vi "NI DOCO DEMO_Same Sample_OK.vi"() -> ()   [LabVIEW 2018]
uses:
  <vilib>/DAQmx/write.llb/DAQmx Write (Digital 1D Wfm NChan NSamp).vi
  <vilib>/DAQmx/write.llb/DAQmx Write (Analog 1D Wfm NChan NSamp).vi
  <vilib>/DAQmx/create/channels.llb/DAQmx Create Channel (AO-Voltage-Basic).vi
  <vilib>/DAQmx/configure/timing.llb/DAQmx Timing (Sample Clock).vi
  <vilib>/Waveform/WDTOps.llb/WDT Number of Waveform Samples DBL.vi
  <vilib>/Waveform/WDTOps.llb/WDT Append Waveforms DBL.vi
  <vilib>/DAQmx/miscellaneous.llb/DAQmx Fill In Error Info.vi
  <vilib>/Waveform/DTblOps.llb/DTbl Digital to Boolean Array.vi
  <vilib>/DAQmx/create/channels.llb/DAQmx Create Channel (DO-Digital Output).vi
  <vilib>/Waveform/DWDTOps.llb/DWDT Uncompress Digital.vi
  <vilib>/Waveform/DWDTOps.llb/DWDT Append Digital Samples.vi
  <resource>/objmgr/daqmx.rc
panel:
  out "DO size 3":i32
  out "DO size 2":i32
  out "DO size":i32
  out "number of samples 3":i32
  out "number of samples 2":i32
  out "number of samples":i32
  out "Mixed Signal Graph 2":cluster{waveform(dbl)[], digitalwaveform[]}(graph)
  out "Mixed Signal Graph":cluster{waveform(dbl)[], digitalwaveform[]}(graph)
  out "initialized array":digitalwaveform[](array[waveform])
  out "Waveform Graph":waveform(dbl)[](graph)
  out "Digital Waveform Graph":digitalwaveform[](graph)
  out "size(s) 4":i32
  out "size(s) 3":i32
  out "size(s) 2":i32
  out "size(s)":i32
  out "NumChans 2":u32
  out "NumChans":u32
  out "Numeric":u32
  in  "Enum":enum16{"A A", "A B", "B B", "B A"}(ring)=enum."A B"
  in  "stop 2":bool
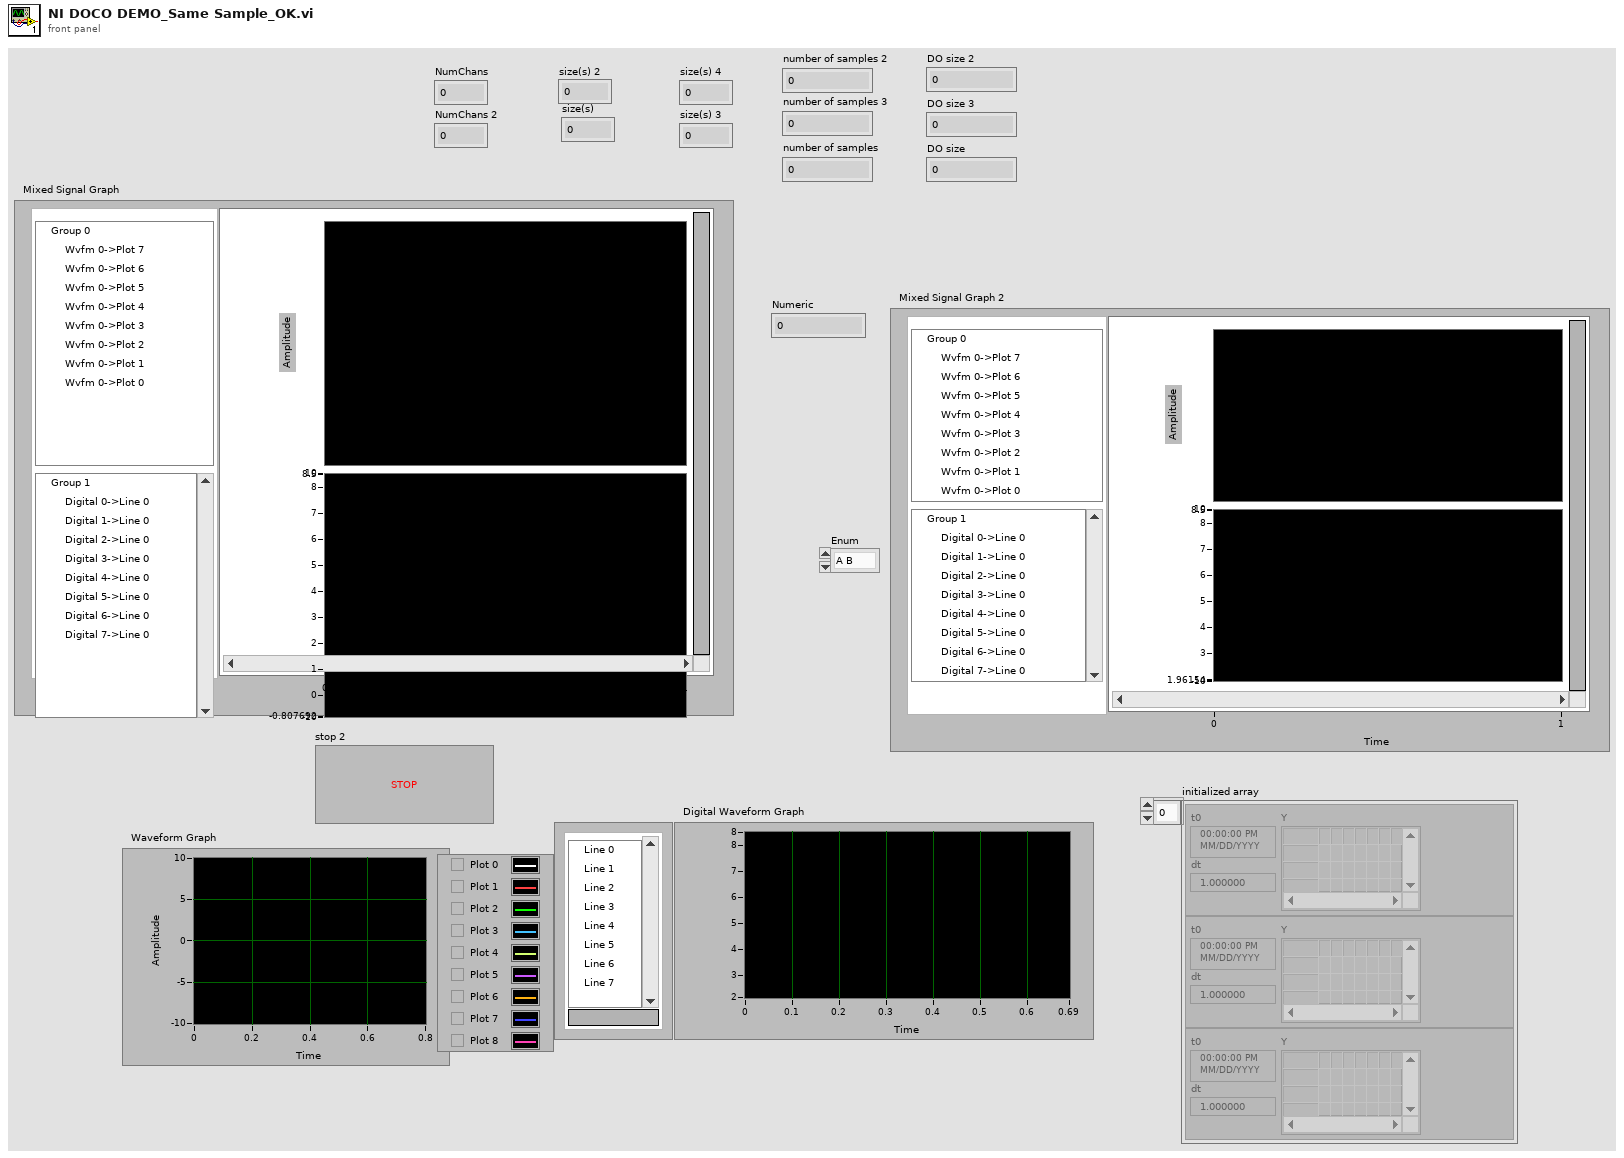
[diagram p1: front panel]
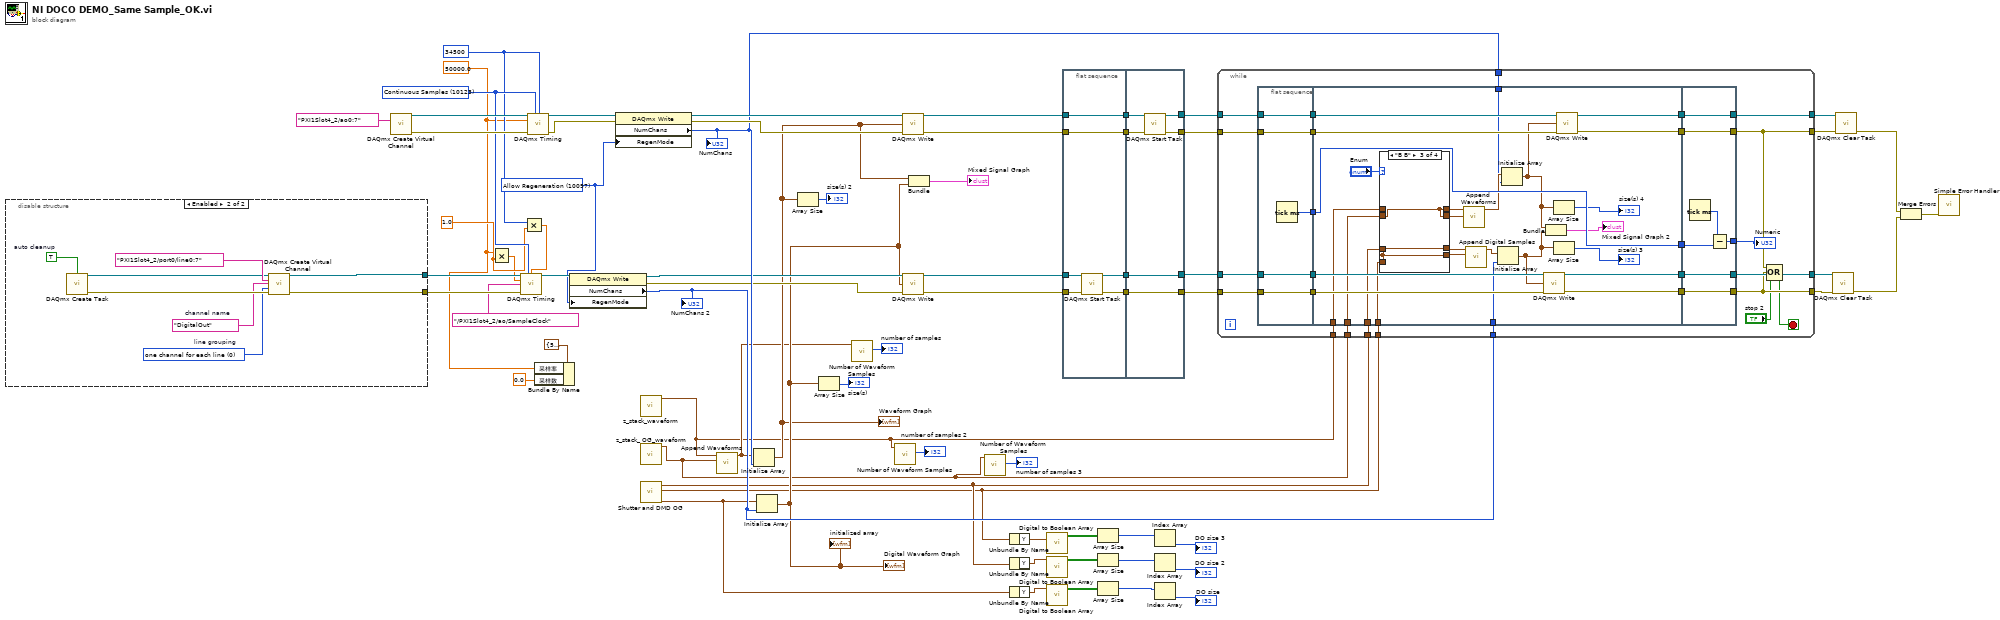
[diagram p0: block diagram]
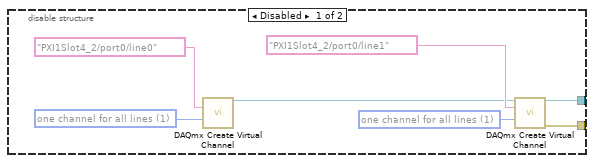
[diagram p2: hidden frame]
diagram:
  w27 = 1.0 ("y")
  w30 = 10097 items=["Allow Regeneration"=10097, "Do Not Allow Regeneration"=10158] ("RegenMode")
  w29 = 34500 ("samples per channel")
  w64 = 10123 items=["Finite Samples"=10178, "Continuous Samples"=10123, "Hardware Timed Single Point"=12522] ("sample mode")
  w2 = 50000.0 ("rate")
  n1 = disable-structure shown="Enabled" {
    disable-tunnel: [w75 w77] -> w66
    disable-tunnel: [w74 w78] -> w65
    frame Disabled {
      w70 = 1 items=["one channel for each line", "one channel for all lines"] ("line grouping")
      w73 = 1 items=["one channel for each line", "one channel for all lines"] ("line grouping")
      n2 = call-poly <vilib>:"DAQmx Create Virtual Channel.vi"("lines"=tag "PXI1Slot4_2/port0/line0", "line grouping"=w70) -> ("task out"=w71:refnum<k21>)  [unwired: 12 in, 1 out]
      n3 = call-poly <vilib>:"DAQmx Create Virtual Channel.vi"("task in"=w71, "lines"=tag "PXI1Slot4_2/port0/line1", "line grouping"=w73) -> ("task out"=w74:refnum<k21>, "error out"=w75:errorcluster)  [unwired: 11 in]
    }
    frame Enabled {
      w79 = TRUE  # auto cleanup
      w83 = 0 items=["one channel for each line", "one channel for all lines"]  # line grouping
      w82 = "DigitalOut"  # channel name
      n4 = call <vilib>:"DAQmx Create Task.vi"("auto cleanup"=w79) -> ("task out"=w80:refnum<k21>, "error out"=w84:errorcluster)  [unwired: 13 in]
      n5 = call-poly <vilib>:"DAQmx Create Virtual Channel.vi"("task in"=w80, "lines"=tag "PXI1Slot4_2/port0/line0:7", "name to assign"=w82, "line grouping"=w83, "error in"=w84) -> ("task out"=w78:refnum<k21>, "error out"=w77:errorcluster)  [unwired: 9 in]
    }
  }
  n6 = call-poly <vilib>:"DAQmx Create Virtual Channel.vi"("physical channels"=tag "PXI1Slot4_2/ao0:7") -> ("task out"=w68:refnum<k21>, "error out"=w67:errorcluster)  [unwired: 13 in]
  n7 = Multiply(x=w2, y=w27) -> (x*y=w4:dbl)
  n8 = Multiply(x=w29, y=w27) -> (x*y=w28:dbl)
  n9 = call-poly <vilib>:"DAQmx Timing.vi"("task/channels in"=w65, "sample mode"=w64, "samples per channel"=w28, "rate"=w4, "source"=tag "/PXI1Slot4_2/ao/SampleClock", "error in"=w66) -> ("task out"=w38:refnum<k21>)  [unwired: 8 in, 1 out]
  n10 = call-poly <vilib>:"DAQmx Timing.vi"("task/channels in"=w68, "sample mode"=w64, "samples per channel"=w29, "rate"=w2, "error in"=w67) -> ("task out"=w43:refnum<k21>, "error out"=w42:errorcluster)  [unwired: 9 in]
  n11 = Bundle By Name(cluster=cluster{"采样率":dbl, "采样数":dbl} {"采样率"=500000.0, "采样数"=130000.0} ("Z stack acquisition 采样信息"), "采样率"=w2, "采样数"=0.0) -> ()  [unwired: 1 out]
  n12 = property class="DAQmx Write"(reference=w38, "RegenMode"=w30) -> (reference out=w37:refnum<k21>, error out=w36:errorcluster, "NumChans"=w35:u32)  [unwired: 1 in]
  "NumChans 2" <- w35
  n13 = property class="DAQmx Write"(reference=w43, error in=w42, "RegenMode"=w30) -> (reference out=w41:refnum<k21>, error out=w40:errorcluster, "NumChans"=w39:u32)
  "NumChans" <- w39
  n14 = call "z_stack_waveform.vi"() -> ("waveform out"=w23:waveform(dbl))  [unwired: 9 in, 2 out]
  n15 = call "z_stack_ OG_waveform.vi"() -> ("waveform out"=w21:waveform(dbl))  [unwired: 15 in, 4 out]
  n16 = call "Shutter and DMD OG.vi"() -> ("output waveform"=w19:digitalwaveform, "output waveform 2"=w9:digitalwaveform, "output waveform1"=w10:digitalwaveform)  [unwired: 8 in]
  n17 = call-poly <vilib>:"Append Waveforms.vi"("waveform B"=w21, "waveform A"=w23) -> ("waveform out"=w24:waveform(dbl))  [unwired: 8 in, 1 out]
  n18 = Initialize Array(w24, w39) -> (w26:waveform(dbl)[])
  "Waveform Graph" <- w26
  n19 = Initialize Array(w19, w35) -> (w32:digitalwaveform[])
  "Digital Waveform Graph" <- w32
  "initialized array" <- w32
  n20 = Array Size(array=w26) -> (size(s)=→"size(s) 2":i32)
  n21 = Array Size(array=w32) -> (size(s)=→"size(s)":i32)
  n22 = call-poly <vilib>:"Number of Waveform Samples.vi"("waveform in"=w24) -> ("number of samples"=→"number of samples":i32)  [unwired: 8 in, 2 out]
  n23 = call-poly <vilib>:"Number of Waveform Samples.vi"("waveform in"=w23) -> ("number of samples"=→"number of samples 2":i32)  [unwired: 8 in, 2 out]
  n24 = call-poly <vilib>:"DAQmx Write.vi"("task/channels in"=w41, "data"=w26, "error in"=w40) -> ("task out"=w62:refnum<k21>, "error out"=w58:errorcluster)  [unwired: 10 in, 1 out]
  n25 = call-poly <vilib>:"DAQmx Write.vi"("task/channels in"=w37, "data"=w32, "error in"=w36) -> ("task out"=w45:refnum<k21>, "error out"=w44:errorcluster)  [unwired: 10 in, 1 out]
  n26 = Bundle(w26, w32) -> (→"Mixed Signal Graph":cluster{waveform(dbl)[], digitalwaveform[]})  [unwired: 1 in]
  n27 = call-poly <vilib>:"Number of Waveform Samples.vi"("waveform in"=w21) -> ("number of samples"=→"number of samples 3":i32)  [unwired: 8 in, 2 out]
  n28 = Unbundle By Name(w9) -> ("Y"=w13:digitaldata)
  n29 = Unbundle By Name(w10) -> ("Y"=w11:digitaldata)
  n30 = Unbundle By Name(w19) -> ("Y"=w14:digitaldata)
  n31 = call-poly <vilib>:"Digital to Boolean Array.vi"("digital data"=w13) -> ("boolean array"=w8:bool[][])  [unwired: 9 in, 1 out]
  n32 = call-poly <vilib>:"Digital to Boolean Array.vi"("digital data"=w11) -> ("boolean array"=w7:bool[][])  [unwired: 9 in, 1 out]
  n33 = call-poly <vilib>:"Digital to Boolean Array.vi"("digital data"=w14) -> ("boolean array"=w18:bool[][])  [unwired: 9 in, 1 out]
  n34 = flat-sequence {
    tunnel: w62 -> [w90]
    tunnel: w45 -> [w89]
    tunnel: w44 -> [w88]
    tunnel: [w90] -> w61
    tunnel: [w87] -> w60
    tunnel: [w86] -> w59
    tunnel: w58 -> [w85]
    tunnel: [w85] -> w57
    tunnel: w61 -> [w94]
    tunnel: [w96] -> w54
    tunnel: w60 -> [w96]
    tunnel: [w95] -> w53
    tunnel: w59 -> [w95]
    tunnel: [w93] -> w56
    tunnel: w57 -> [w92]
    tunnel: [w91] -> w55
    frame #0 {
      n35 = call <vilib>:"DAQmx Start Task.vi"("task/channels in"=w89, "error in"=w88) -> ("task out"=w87:refnum<k21>, "error out"=w86:errorcluster)  [unwired: 12 in]
    }
    frame #1 {
      n36 = call <vilib>:"DAQmx Start Task.vi"("task/channels in"=w94, "error in"=w92) -> ("task out"=w93:refnum<k21>, "error out"=w91:errorcluster)  [unwired: 12 in]
    }
  }
  n37 = Array Size(array=w8) -> (size(s)=w6:i32[])
  n38 = Array Size(array=w7) -> (size(s)=w5:i32[])
  n39 = Array Size(array=w18) -> (size(s)=w17:i32[])
  n40 = Index Array(array=w6) -> (element=→"DO size 3":i32)  [unwired: 1 in]
  n41 = Index Array(array=w5) -> (element=→"DO size 2":i32)  [unwired: 1 in]
  n42 = Index Array(array=w17) -> (element=→"DO size":i32)  [unwired: 1 in]
  n43 = while {
    tunnel: w56 -> [w121]
    tunnel: w55 -> [w120]
    tunnel: w54 -> [w123]
    tunnel: w53 -> [w122]
    tunnel: [w117] -> w51
    tunnel: [w119] -> w52
    tunnel: [w118] -> w50
    tunnel: [w116] -> w49
    tunnel: w23 -> [w113]
    tunnel: w21 -> [w112]
    tunnel: w10 -> [w111]
    tunnel: w9 -> [w110]
    tunnel: w39 -> [w98]
    tunnel: w35 -> [w97]
    stop <- w115 stop-if-true
    n44 = flat-sequence {
      tunnel: w120 -> [w125]
      tunnel: w121 -> [w126]
      tunnel: w122 -> [w127]
      tunnel: w123 -> [w128]
      tunnel: [w128] -> w109
      tunnel: [w127] -> w108
      tunnel: [w126] -> w107
      tunnel: [w125] -> w106
      tunnel: [w124] -> w101
      tunnel: w113 -> [w146]
      tunnel: w112 -> [w145]
      tunnel: w111 -> [w144]
      tunnel: w110 -> [w143]
      tunnel: w109 -> [w155]
      tunnel: w108 -> [w154]
      tunnel: w107 -> [w153]
      tunnel: w106 -> [w152]
      tunnel: [w151] -> w105
      tunnel: [w150] -> w104
      tunnel: [w149] -> w103
      tunnel: [w148] -> w102
      tunnel: w101 -> [w138]
      tunnel: [w138] -> w100
      tunnel: w98 -> [w136]
      tunnel: w97 -> [w134]
      tunnel: [w171] -> w116
      tunnel: [w172] -> w117
      tunnel: [w173] -> w118
      tunnel: [w174] -> w119
      tunnel: w105 -> [w174]
      tunnel: w104 -> [w173]
      tunnel: w103 -> [w172]
      tunnel: w102 -> [w171]
      tunnel: w100 -> [w169]
      tunnel: [w168] -> w99
      frame #0 {
        n45 = Tick Count (ms)() -> (millisecond timer value=w124:u32)
      }
      frame #1 {
        n46 = case shown="\"B B\"" "Enum" {
          tunnel: w146 -> [w157 w161 _ w166]
          tunnel: w145 -> [_ w160 w163 w167]
          tunnel: w144 -> [w156 w159 _ w164]
          tunnel: w143 -> [_ w158 w162 w165]
          tunnel: [w157 w161 w163 w167] -> w142
          tunnel: [w157 w160 w163 w166] -> w141
          tunnel: [w156 w159 w162 w165] -> w140
          tunnel: [w156 w158 w162 w164] -> w139
          frame "A A", Default {
          }
          frame "A B" {
          }
          frame "B B" {
          }
          frame "B A" {
          }
        }
        n47 = call-poly <vilib>:"Append Waveforms.vi"("waveform B"=w141, "waveform A"=w142) -> ("waveform out"=w137:waveform(dbl))  [unwired: 8 in, 1 out]
        n48 = call-poly <vilib>:"Append Digital Samples.vi"("digital waveform B"=w139, "digital waveform A"=w140) -> ("digital waveform out"=w135:digitalwaveform)  [unwired: 8 in, 1 out]
        n49 = Initialize Array(w135, w134) -> (w132:digitalwaveform[])
        n50 = Initialize Array(w137, w136) -> (w133:waveform(dbl)[])
        n51 = call-poly <vilib>:"DAQmx Write.vi"("task/channels in"=w155, "data"=w132, "error in"=w154) -> ("task out"=w150:refnum<k21>, "error out"=w148:errorcluster)  [unwired: 10 in, 1 out]
        n52 = Bundle(w133, w132) -> (→"Mixed Signal Graph 2":cluster{waveform(dbl)[], digitalwaveform[]})  [unwired: 1 in]
        n53 = Array Size(array=w133) -> (size(s)=→"size(s) 4":i32)
        n54 = Array Size(array=w132) -> (size(s)=→"size(s) 3":i32)
        n55 = call-poly <vilib>:"DAQmx Write.vi"("task/channels in"=w153, "data"=w133, "error in"=w152) -> ("task out"=w151:refnum<k21>, "error out"=w149:errorcluster)  [unwired: 10 in, 1 out]
      }
      frame #2 {
        n56 = Tick Count (ms)() -> (millisecond timer value=w170:u32)
        n57 = Subtract(x=w170, y=w169) -> (x-y=w168:u32)
      }
    }
    n58 = Compound Arithmetic op=OR(w117, w116, "stop 2") -> (w115:bool)
    "Numeric" <- w99
  }
  n59 = call <vilib>:"DAQmx Clear Task.vi"("task in"=w50, "error in"=w49) -> ("error out"=w47:errorcluster)  [unwired: 13 in]
  n60 = call <vilib>:"DAQmx Clear Task.vi"("task in"=w52, "error in"=w51) -> ("error out"=w48:errorcluster)  [unwired: 13 in]
  n61 = Merge Errors(w48, w47) -> (w46:errorcluster)
  n62 = call <vilib>:"Simple Error Handler.vi"("error in (no error)"=w46) -> ()  [unwired: 4 in, 5 out]
